vi "Add Node.vi"(11 "Abstract Graph in":refnum<class "Abstract Graph.lvclass">) -> (3 "Abstract Graph out":refnum<class "Abstract Graph.lvclass">)   [LabVIEW 2021, in "GraphLib.lvlib" / "Abstract Graph.lvclass"]
uses:
  Abstract Graph.lvclass
  Abstract Graph.lvclass/Abstract Graph.ctl
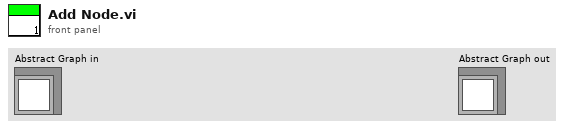
[diagram p1: front panel]
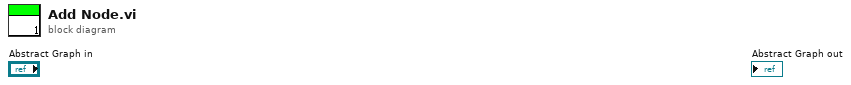
[diagram p0: block diagram]
diagram:
